vi "CalcVandA.vi"(0 "distance":i32, 1 "fps":sgl) -> (2 "Accel":dbl, 3 "Velocity":dbl, 4 "BKPT shift":i32)   [LabVIEW 2022 SP3]
panel:
  out "vel calc":dbl=240000.0
  out "accel calc":dbl=22000000.0
  in  "vel upper limit":dbl=400000.0
  in  "accel upper limit":dbl=40000000.0
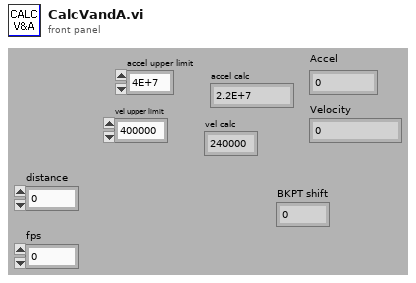
[diagram p1: front panel]
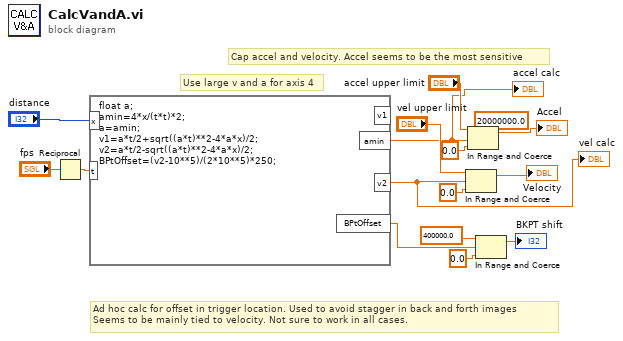
[diagram p0: block diagram]
diagram:
  (unwired) 20000000.0 ("Accel")
  # "Ad hoc calc for offset in trigger location. Used to avoid stagger in back and forth images\nSeems to be mainly tied to velocity. Not sure to work in all cases."
  # "Cap accel and velocity. Accel seems to be the most sensitive"
  # "Use large v and a for axis 4"
  n1 = Reciprocal(x="fps") -> (1/x=w10:sgl)
  n2 = formula code="float a;\namin=4*x/(t*t)*2;\na=amin;\nv1=a*t/2+sqrt((a*t)**2-4*a*x)/2;\nv2=a*t/2-sqrt((a*t)**2-4*a*x)/2;\nBPtOffset=(v2-10**5)/(2*10**5)*250;"("x"="distance", "t"=w10) -> ("v2"=w2:dbl, "amin"=w3:dbl, "BPtOffset"=w7:dbl)  [unwired: 1 out]
  "accel calc" <- w3
  "vel calc" <- w2
  n3 = In Range and Coerce(upper limit="vel upper limit", x=w2, lower limit=0.0) -> (coerced(x)=→"Velocity":dbl)  [unwired: 1 out]
  n4 = In Range and Coerce(upper limit="accel upper limit", x=w3, lower limit=0.0) -> (coerced(x)=→"Accel":dbl)  [unwired: 1 out]
  n5 = In Range and Coerce(upper limit=400000.0, x=w7, lower limit=0.0) -> (coerced(x)=→"BKPT shift":dbl)  [unwired: 1 out]
